vi "Vin_DC2ch.vi"(2 "Fondo Scala AI1":dbl(ring)=10.0 items=["10"=10.0, "5"=5.0, "0.5"=0.5, "0.05"=0.05], 3 "Fondo Scala AI0":dbl(ring)=10.0 items=["10"=10.0, "5"=5.0, "0.5"=0.5, "0.05"=0.05]) -> (0 "V_in(Volt)":dbl=0.052760983012389205 format="%.3f", 1 "Corrente (mA)":dbl=0.052760983012389205 format="%.4f")   [LabVIEW 2014]
doc: "Vin 2ch\nlwgge due canali con fondo scala regolabile\nVers. per 8.6\nnov 2013"
uses:
  <vilib>/DAQmx/read.llb/DAQmx Read (Analog 2D DBL NChan NSamp).vi
  <vilib>/Analysis/baseanly.llb/Mean (DBL).vi
  <vilib>/DAQmx/create/channels.llb/DAQmx Create Channel (AI-Voltage-Basic).vi
  <vilib>/DAQmx/configure/timing.llb/DAQmx Timing (Sample Clock).vi
  <vilib>/DAQmx/miscellaneous.llb/DAQmx Fill In Error Info.vi
  <vilib>/Analysis/NI_AALBase.lvlib
panel:
  in  "Resistenza":dbl=2.7 max=100000.0
  # "1) Scegliere il fondo scala dell'analog input: \n[10, 5, 0.5, 0.05] per la 6024"
  # "2) Premere la freccia bianca del menu"
  # "3) Tensione misurata sul CB33"
  # "4) Tensione misurata sul CB68"
  # "Collegare la massa del breadboard\nalla massa (CB29)"
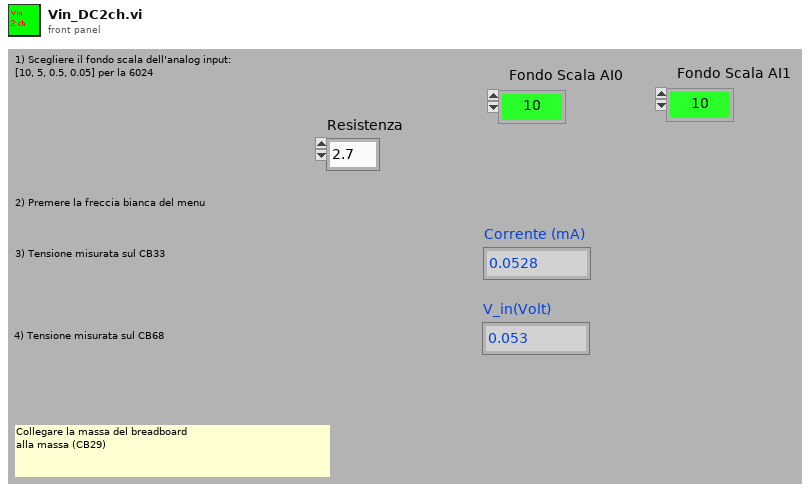
[diagram p1: front panel]
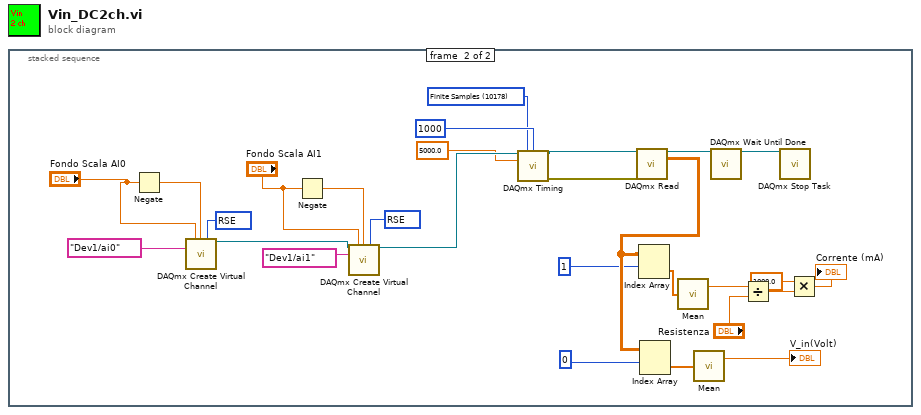
[diagram p0: block diagram]
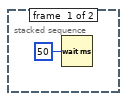
[diagram p2: hidden frame]
diagram:
  n1 = stacked-sequence {
    frame #0 {
      n2 = Wait (ms)(milliseconds to wait=u32 50) -> ()  [unwired: 1 out]
    }
    frame #1 {
      w10 = 10083 items=["default"=-1, "RSE"=10083, "NRSE"=10078, "Differential"=10106, "Pseudodifferential"=12529] ("input terminal configuration")
      w20 = 10178 items=["Finite Samples"=10178, "Continuous Samples"=10123, "Hardware Timed Single Point"=12522] ("sample mode")
      w28 = 10083 items=["default"=-1, "RSE"=10083, "NRSE"=10078, "Differential"=10106, "Pseudodifferential"=12529] ("input terminal configuration")
      n3 = Negate(x="Fondo Scala AI0") -> (-x=w11:dbl)
      n4 = call-poly <vilib>:"DAQmx Create Virtual Channel.vi"("maximum value"="Fondo Scala AI0", "minimum value"=w11, "input terminal configuration"=w10, "physical channels"=tag "Dev1/ai0") -> ("task out"=w8:refnum<k21>)  [unwired: 5 in, 6 out]
      n5 = Negate(x="Fondo Scala AI1") -> (-x=w29:dbl)
      n6 = call-poly <vilib>:"DAQmx Create Virtual Channel.vi"("task in"=w8, "maximum value"="Fondo Scala AI1", "minimum value"=w29, "input terminal configuration"=w28, "physical channels"=tag "Dev1/ai1") -> ("task out"=w23:refnum<k21>)  [unwired: 4 in, 6 out]
      n7 = call-poly <vilib>:"DAQmx Timing.vi"("task/channels in"=w23, "sample mode"=w20, "samples per channel"=u32 1000, "rate"=5000.0) -> ("task out"=w26:refnum<k21>, "error out"=w25:errorcluster)  [unwired: 3 in, 7 out]
      n8 = call-poly <vilib>:"DAQmx Read.vi"("task/channels in"=w26, "error in"=w25) -> ("task out"=w21:refnum<k21>, "data"=w17:dbl[][])  [unwired: 1 in, 11 out]
      n9 = Index Array(array=w17, index (row)=1) -> (element=w15:dbl[])  [unwired: 1 in]
      n10 = Index Array(array=w17, index (row)=0) -> (element=w14:dbl[])  [unwired: 1 in]
      n11 = call-poly <vilib>:"Mean.vi"("X"=w15) -> ("mean"=w18:dbl)  [unwired: 1 out]
      n12 = call-poly <vilib>:"Mean.vi"("X"=w14) -> ("mean"=→"V_in(Volt)":dbl)  [unwired: 1 out]
      n13 = call <vilib>:"DAQmx Wait Until Done.vi"("task/channels in"=w21) -> ("task out"=w19:refnum<k21>)  [unwired: 2 in, 12 out]
      n14 = Divide(x=w18, y="Resistenza") -> (x/y=w5:dbl)
      n15 = call <vilib>:"DAQmx Stop Task.vi"("task/channels in"=w19) -> ()  [unwired: 1 in, 14 out]
      n16 = Multiply(x=1000.0, y=w5) -> (x*y=→"Corrente (mA)":dbl)
    }
  }
